vi "New Client.vi"   [LabVIEW 2020, in "WAMP Client.lvclass"]
uses:
  <userlib>/lvwamp/WAMP Client/WAMP Client.lvclass
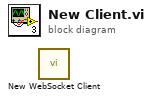
[diagram p0: block diagram]
diagram:
  n1 = call <userlib>:"New WebSocket Client.vi"() -> ()  [unwired: 14 in, 2 out]
